vi "MFLI Initialize module.vi"(10 "module Id":T5=1 items=["sweep", "scopeModule", "dataAcquisitionModule", "pidAdvisor", "awgModule", "impedanceModule", "multiDeviceSyncModule", "zoomFFT", "trigger", "deviceSettings", "record", "precompensationAdvisor"], 11 "ACQ  status in":T1 {"ModuleHandles"."ModHandle" format="0x%08x"; "ModuleHandles"."Conn" format="0x%08x"; "Lock-in Handle"."Handle" format="0x%08x"; "Lock-in Handle"."Conn" format="0x%08x"}) -> (0 "Error Out":errorcluster, 3 "ACQ  status out":T1 {"ModuleHandles"."ModHandle" format="0x%08x"; "ModuleHandles"."Conn" format="0x%08x"; "Lock-in Handle"."Handle" format="0x%08x"; "Lock-in Handle"."Conn" format="0x%08x"})   [LabVIEW 2022 SP3, in "Lock-in module.lvlib"]
uses:
  Lock-in module.lvlib
  <instrlib>/Zurich Instruments LabOne/Public/Modules/ziTypeModEnum.ctl
  ctl/ACQ status.ctl
  <instrlib>/Zurich Instruments LabOne/Public/ziTypeHandle.ctl
  <instrlib>/Zurich Instruments LabOne/Public/Modules/ziTypeModHandle.ctl
  ctl/ACQ info.ctl
  <instrlib>/Zurich Instruments LabOne/Zurich Instruments LabOne.lvlib
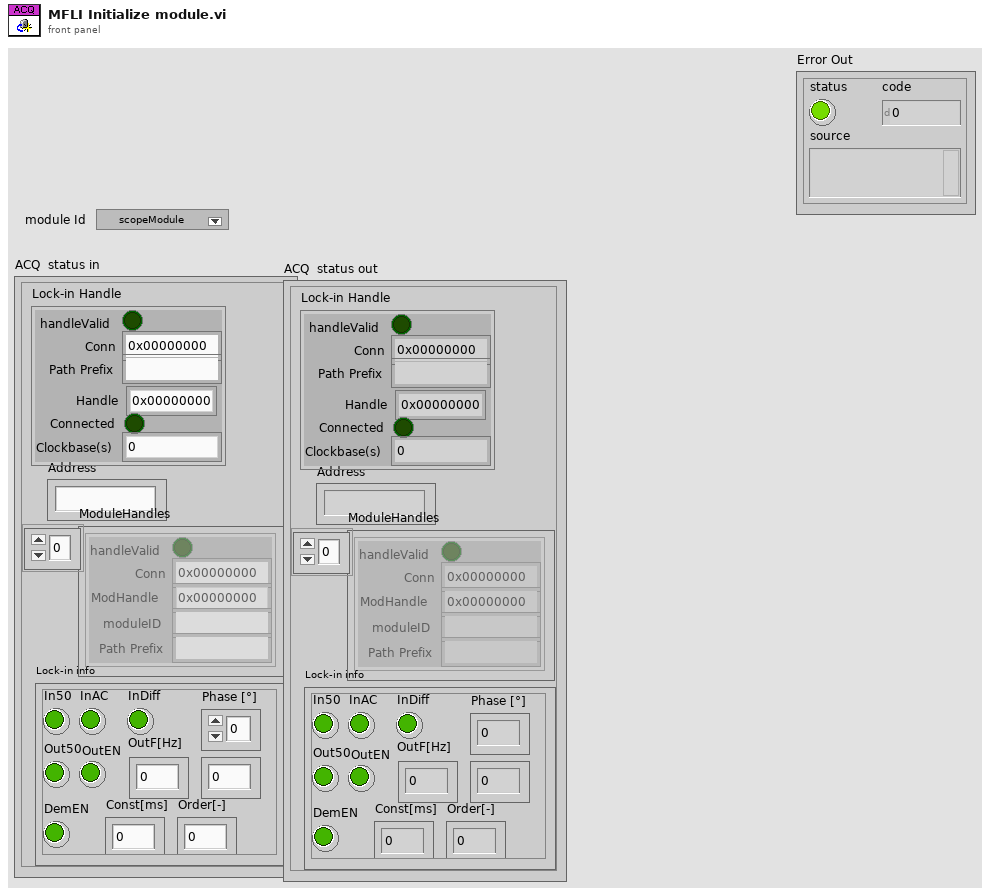
[diagram p1: front panel]
types:
  T1 = typedef "Lock-in module.lvlib/ACQ status.ctl" = cluster{"Lock-in Handle":T2, "Address":string, "ModuleHandles":T3[], "Lock-in info":T4}
  T2 = typedef "Zurich Instruments LabOne.lvlib/ziTypeHandle.ctl" = cluster{"handleValid":bool, "Conn":u64, "Path Prefix":string, "Handle":u64, "Connected":bool, "Clockbase(s)":dbl}
  T3 = typedef "Zurich Instruments LabOne.lvlib/ziTypeModHandle.ctl" = cluster{"handleValid":bool, "Conn":u64, "ModHandle":u64, "moduleID":string, "Path Prefix":string}
  T4 = typedef "Lock-in module.lvlib/ACQ info.ctl" = cluster{"In50":bool, "InAC":bool, "InDiff":bool, "Out50":bool, "OutEN":bool, "OutF[Hz]":dbl, "OutA[V]":dbl, "DemEN":bool, "Const[ms]":dbl, "Order[-]":i32, "Phase [°]":dbl}
  T5 = typedef "Zurich Instruments LabOne.lvlib/ziTypeModEnum.ctl" = u16
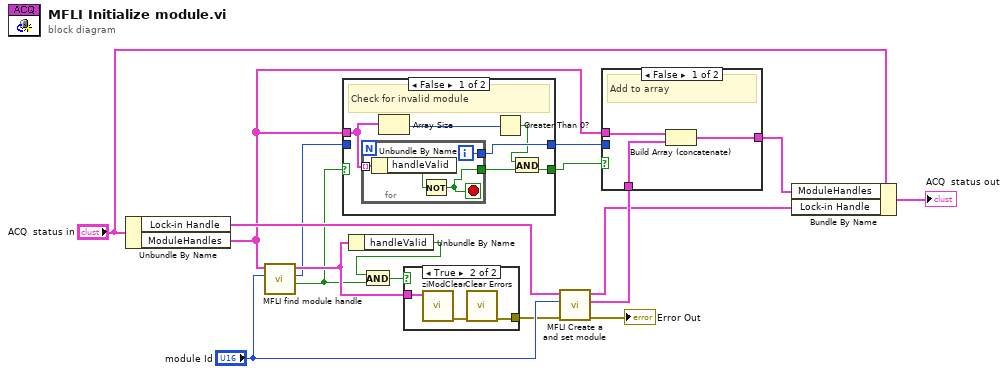
[diagram p0: block diagram]
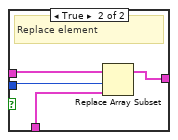
[diagram p4: hidden frame]
diagram:
  n1 = Unbundle By Name("ACQ  status in") -> ("Lock-in Handle"=w17:T2, "ModuleHandles"=w5:T3[])
  n2 = call "MFLI find module handle.vi"("module Id"="module Id", "ModuleHandles"=w5) -> ("was found"=w9:bool, "index"=w8:i32, "ziModHandle out"=w12:T3)  [unwired: 7 in]
  n3 = case shown="False" w9 {
    selector: w9 -> [_ w29]
    tunnel: w8 -> [_ w28]
    tunnel: [w19 w29] -> w6
    tunnel: [w21 w28] -> w7
    tunnel: w5 -> [w22 _]
    frame False {
      # "Check for invalid module"
      n4 = for {
        tunnel: w22 -> [w27] mode=indexing
        tunnel: [w26] -> w21
        tunnel: [w24] -> w23
        i -> [w26]
        stop <- w24 stop-if-true
        n5 = Unbundle By Name(w27) -> ("handleValid"=w25:bool)
        n6 = Not(x=w25) -> (.not. x?=w24:bool)
      }
      n7 = Array Size(array=w22) -> (size(s)=w20:i32)
      n8 = Greater Than 0?(x=w20) -> (x > 0?=w18:bool)
      n9 = And(x=w18, y=w23) -> (x .and. y?=w19:bool)
    }
    frame True {
    }
  }
  n10 = Unbundle By Name(w12) -> ("handleValid"=w14:bool)
  n11 = And(x=w14, y=w9) -> (x .and. y?=w13:bool)
  n12 = case shown="True" w13 {
    tunnel: w12 -> [_ w32]
    tunnel: [_ w30] -> w10
    frame False {
    }
    frame True {
      n13 = call <instrlib>:"ziModClear.vi"("ziModHandle In"=w32) -> ("Error Out"=w31:errorcluster)  [unwired: 8 in, 1 out]
      n14 = call <vilib>:"Clear Errors.vi"("error in (no error)"=w31) -> ("error out"=w30:errorcluster)  [unwired: 5 in, 1 out]
    }
  }
  n15 = call "MFLI Create a and set module.vi"("error in (no error)"=w10, "module Id"="module Id", "Lock-in Handle"=w17) -> ("Error Out"=→"Error Out":errorcluster, "ModHandle Out"=w2:T3, "Lock-in Handle out"=w1:T2)  [unwired: 6 in]
  n16 = case shown="False" w6 {
    tunnel: [w35 w38] -> w4
    tunnel: w5 -> [w34 w39]
    tunnel: w2 -> [w33 w36]
    tunnel: w7 -> [_ w37]
    frame False {
      # "Add to array"
      n17 = Build Array (concatenate)(w34, w33) -> (w35:T3[])
    }
    frame True {
      # "Replace element"
      n18 = Replace Array Subset(array=w39, new element=w36, index=w37) -> (w38:T3[])
    }
  }
  n19 = Bundle By Name(cluster="ACQ  status in", "ModuleHandles"=w4, "Lock-in Handle"=w1) -> (→"ACQ  status out":T1)
